vi "Newport ITX-D3N GET DewPoint Data.vi"(7 "iTHX Commands":T1="*SRTF", 8 "Error In":errorcluster, 11 "TCP Network Connection In":refnum<k5>) -> (0 "Error Out":errorcluster, 1 "In Range?":bool, 2 "Output Data":dbl, 3 "TCP Network Connection Out":refnum<k5>)   [LabVIEW 2018]
uses:
  Type Definitions/iTHX.ctl
panel:
  out "data out":string
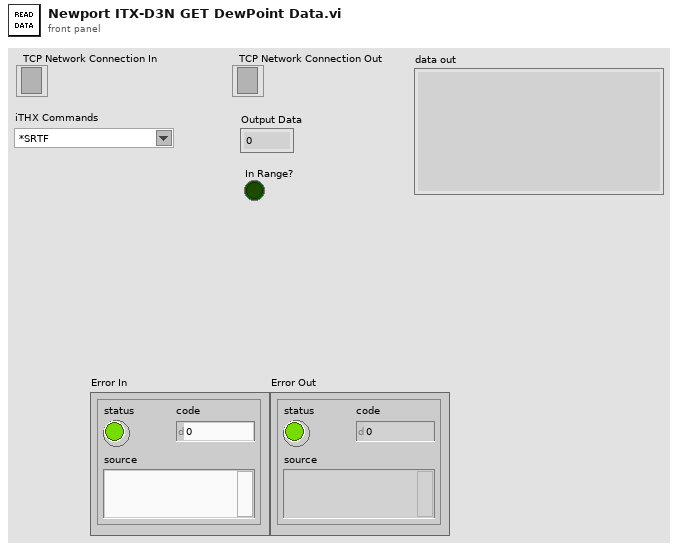
[diagram p1: front panel]
types:
  T1 = typedef "iTHX.ctl" = string
  T2 = enum16{"Standard", "Buffered", "CRLF", "Immediate"}
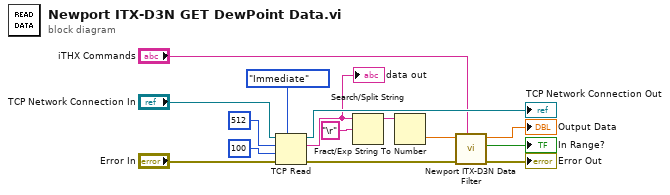
[diagram p0: block diagram]
diagram:
  n1 = TCP Read(connection ID="TCP Network Connection In", bytes to read=512, error in (no error)="Error In", 7:T2."Immediate" ("mode (standard)"), 9:100) -> (connection ID out=→"TCP Network Connection Out":refnum<k5>, data out=w7:string, error out=w5:errorcluster)
  "data out" <- w7
  n2 = Search/Split String(string=w7, search string/char (-)="\r") -> (substring before match=w6:string)  [unwired: 1 in, 2 out]
  n3 = Fract/Exp String To Number(string=w6) -> (number=w3:dbl)  [unwired: 3 in, 1 out]
  n4 = call "Newport ITX-D3N Data Filter.vi"("iTHX Commands"="iTHX Commands", "Error In"=w5, "Current Data"=w3) -> ("Error Out"=→"Error Out":errorcluster, "In Range?"=→"In Range?":bool, "Data Output"=→"Output Data":dbl)  [unwired: 6 in]
